vi "04-RandomNumbers.vi"() -> ()   [LabVIEW 2019]
panel:
  out "Loop Count":dbl
  out "Random Number":dbl
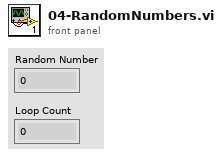
[diagram p1: front panel]
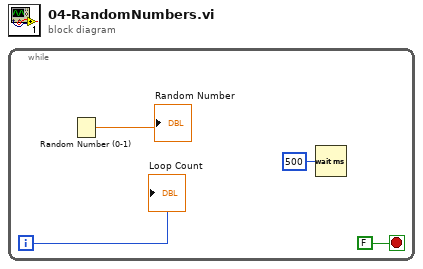
[diagram p0: block diagram]
diagram:
  n1 = while {
    i -> [w4]
    stop <- FALSE stop-if-true
    n2 = Random Number (0-1)() -> (number: 0 to 1=→"Random Number":dbl)
    n3 = Wait (ms)(milliseconds to wait=u32 500) -> ()  [unwired: 1 out]
    "Loop Count" <- w4
  }
